vi "RelativeStimTiming.vi"(0 "stimulus parameters":T1, 1 "time":dbl format="%#_13g") -> (2 "time until next":dbl, 3 "delivered":i32, 4 "remaining":i32)   [LabVIEW 2014]
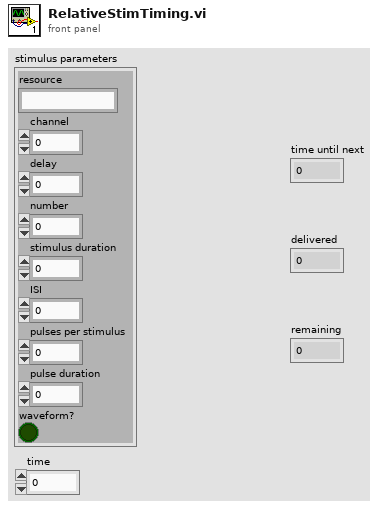
[diagram p1: front panel]
types:
  T1 = cluster{"resource":string, "channel":u16, "delay":dbl, "number":i32, "stimulus duration":dbl, "ISI":dbl, "pulses per stimulus":u16, "pulse duration":dbl, "waveform?":bool}
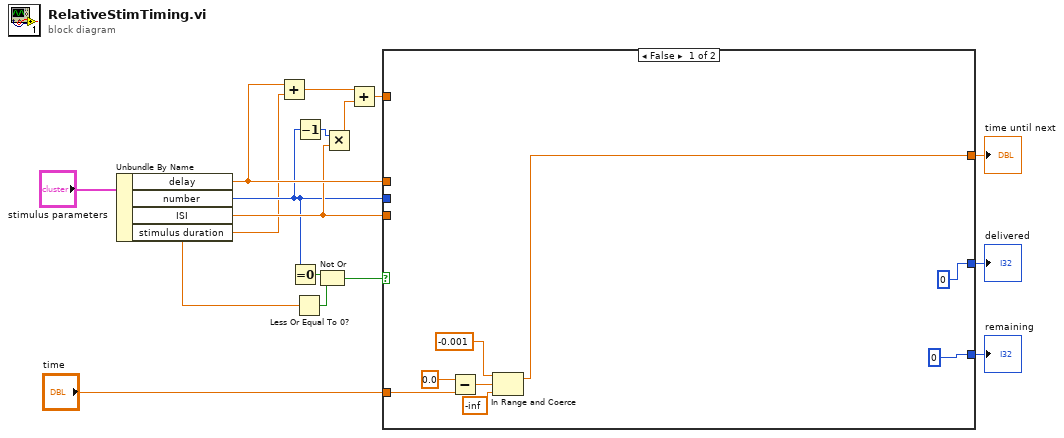
[diagram p0: block diagram]
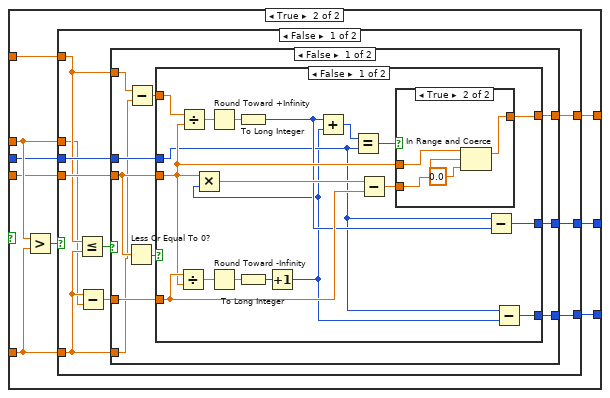
[diagram p2: hidden frame]
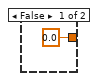
[diagram p3: hidden frame]
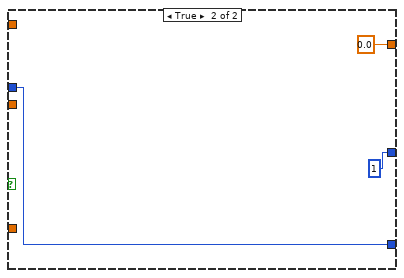
[diagram p4: hidden frame]
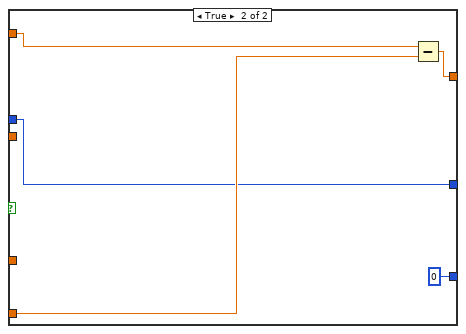
[diagram p5: hidden frame]
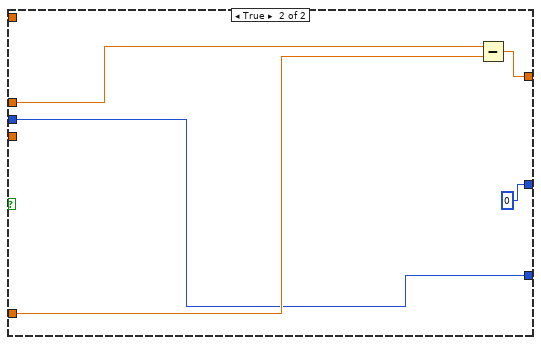
[diagram p6: hidden frame]
diagram:
  n1 = Unbundle By Name("stimulus parameters") -> ("delay"=w4:dbl, "number"=w2:i32, "ISI"=w3:dbl, "stimulus duration"=w1:dbl)
  n2 = Add(x=w4, y=w1) -> (x+y=w7:dbl)
  n3 = Equal To 0?(x=w2) -> (x = 0?=w14:bool)
  n4 = Less Or Equal To 0?(x=w1) -> (x <= 0?=w13:bool)
  n5 = Decrement(x=w2) -> (x-1=w9:i32)
  n6 = Not Or(1:w13, 2:w14) -> (0:w15:bool)
  n7 = Multiply(x=w9, y=w3) -> (x*y=w8:dbl)
  n8 = Add(x=w7, y=w8) -> (x+y=w6:dbl)
  n9 = case shown="False" w15 {
    tunnel: [w18 w30] -> w12
    tunnel: [0 w26] -> w11
    tunnel: [0 w27] -> w10
    tunnel: w6 -> [_ w25]
    tunnel: "time" -> [w22 w31]
    tunnel: w4 -> [_ w32]
    tunnel: w3 -> [_ w28]
    tunnel: w2 -> [_ w29]
    frame False {
      n10 = Subtract(x=0.0, y=w22) -> (x-y=w20:dbl)
      n11 = In Range and Coerce(upper limit=-0.001, x=w20, lower limit=-inf) -> (coerced(x)=w18:dbl)  [unwired: 1 out]
    }
    frame True {
      n12 = Greater?(x=w32, y=w31) -> (0:w33:bool)
      n13 = case shown="False" w33 {
        tunnel: w32 -> [w35 w89]
        tunnel: w31 -> [w36 w88]
        tunnel: [w39 w87] -> w30
        tunnel: w29 -> [w42 w86]
        tunnel: w28 -> [w41 _]
        tunnel: [w37 w86] -> w27
        tunnel: [w38 0] -> w26
        tunnel: w25 -> [w40 _]
        frame False {
          n14 = Less Or Equal?(x=w40, y=w36) -> (x <= y?=w43:bool)
          n15 = Subtract(x=w36, y=w35) -> (x-y=w34:dbl)
          n16 = case shown="False" w43 {
            tunnel: w42 -> [w49 w81]
            tunnel: w41 -> [w48 _]
            tunnel: w36 -> [w45 w83]
            tunnel: w40 -> [w46 w84]
            tunnel: [w52 w82] -> w39
            tunnel: [w51 w81] -> w38
            tunnel: [w50 0] -> w37
            tunnel: w34 -> [w47 _]
            frame False {
              n17 = Less Or Equal To 0?(x=w48) -> (x <= 0?=w53:bool)
              n18 = Subtract(x=w46, y=w45) -> (x-y=w44:dbl)
              n19 = case shown="False" w53 {
                tunnel: [w60 0.0] -> w52
                tunnel: [w58 1] -> w51
                tunnel: [w56 w77] -> w50
                tunnel: w49 -> [w55 w77]
                tunnel: w48 -> [w61 _]
                tunnel: w47 -> [w63 _]
                tunnel: w44 -> [w71 _]
                frame False {
                  n20 = Divide(x=w63, y=w61) -> (x/y=w68:dbl)
                  n21 = Divide(x=w71, y=w61) -> (x/y=w70:dbl)
                  n22 = Round Toward +Infinity(x=w70) -> (ceil(x): smallest int >= x=w69:dbl)
                  n23 = Round Toward -Infinity(1:w68) -> (0:w67:dbl)
                  n24 = To Long Integer(number=w69) -> (32bit integer=w57:i32)
                  n25 = To Long Integer(number=w67) -> (32bit integer=w59:i32)
                  n26 = Increment(x=w59) -> (x+1=w54:i32)
                  n27 = Multiply(x=w61, y=w54) -> (x*y=w64:dbl)
                  n28 = Add(x=w57, y=w54) -> (x+y=w65:i32)
                  n29 = Equal?(x=w65, y=w55) -> (x = y?=w66:bool)
                  n30 = Subtract(x=w64, y=w63) -> (x-y=w62:dbl)
                  n31 = case shown="True" w66 {
                    tunnel: w62 -> [_ w76]
                    tunnel: w61 -> [_ w74]
                    tunnel: [0.0 w73] -> w60
                    frame False {
                    }
                    frame True {
                      n32 = In Range and Coerce(upper limit=w74, x=w76, lower limit=0.0) -> (coerced(x)=w73:dbl)  [unwired: 1 out]
                    }
                  }
                  n33 = Subtract(x=w55, y=w57) -> (x-y=w58:i32)
                  n34 = Subtract(x=w55, y=w54) -> (x-y=w56:i32)
                }
                frame True {
                }
              }
            }
            frame True {
              n35 = Subtract(x=w84, y=w83) -> (x-y=w82:dbl)
            }
          }
        }
        frame True {
          n36 = Subtract(x=w89, y=w88) -> (x-y=w87:dbl)
        }
      }
    }
  }
  "time until next" <- w12
  "delivered" <- w11
  "remaining" <- w10
